vi "Add PV - NT Enum (Reference).vi"(5 "is read only? (F)":bool, 6 "initial timestamp":timestamp, 7 "PV name":string, 8 "error in (no error)":errorcluster, 10 "ref":refnum<vi>, 11 "Server in":refnum<class "Server.lvclass">) -> (0 "error out":errorcluster, 2 "ref out":refnum<vi>, 3 "Server out":refnum<class "Server.lvclass">)   [LabVIEW 2020, in "PV Access.lvlib" / "PVA Server.lvlib" / "Server.lvclass"]
uses:
  Server.lvclass
  Server.lvclass/Server.ctl
  PV Data/NT Enum/NT Enum.lvclass
  Source/Source.lvclass
  PV Data/PV Data.lvlib
  PV Data/NT Enum/Create - Enum.vi
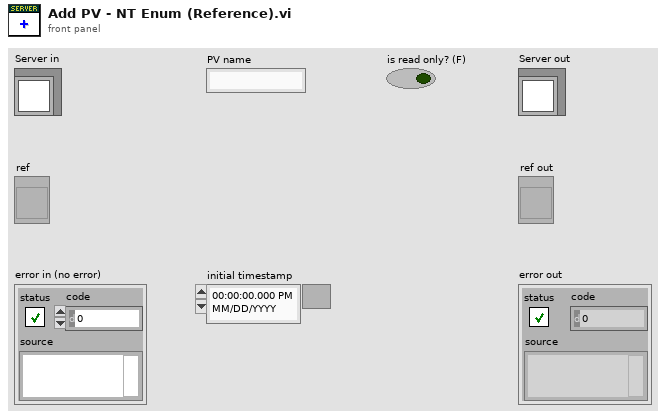
[diagram p1: front panel]
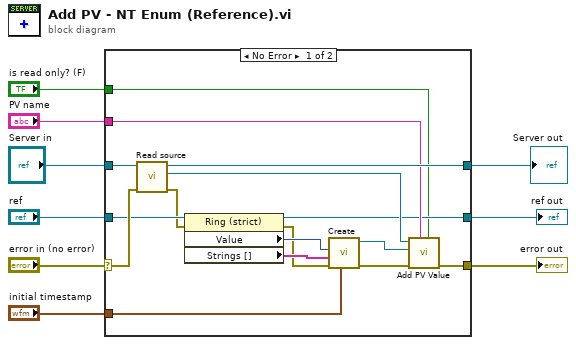
[diagram p0: block diagram]
diagram:
  n1 = case shown="No Error" "error in (no error)" {
    selector: "error in (no error)" -> [w21 w28]
    tunnel: [w20 w28] -> w8
    tunnel: [w24 w27] -> w6
    tunnel: "Server in" -> [w25 w27]
    tunnel: "PV name" -> [w22 _]
    tunnel: "initial timestamp" -> [w17 _]
    tunnel: "ref" -> [w16 w26]
    tunnel: [w11 w26] -> w2
    tunnel: "is read only? (F)" -> [w10 _]
    frame No Error {
      n2 = call "Read source.vi"("error in (no error)"=w21, "Server in"=w25) -> ("error out"=w15:errorcluster, "Source"=w23:refnum<class "Source.lvclass">, "Server out"=w24:refnum<class "Server.lvclass">)  [unwired: 7 in]
      n3 = property class="Ring (strict)"(reference=w16, error in=w15) -> (reference out=w11:refnum<vi>, error out=w12:errorcluster, "Value"=w14:u16, "Strings []"=w13:string[])
      n4 = call-poly "Create.vi"("initial timestamp"=w17, "error in (no error)"=w12, "choices"=w13, "initial index"=w14) -> ("error out"=w19:errorcluster, "NT Enum out"=w18:refnum<class "NT Enum.lvclass">)  [unwired: 6 in]
      n5 = call "Add PV Value.vi"("is read only? (F)"=w10, "PV name"=w22, "error in"=w19, "value in"=w18, "Source in"=w23) -> ("error out"=w20:errorcluster)  [unwired: 4 in, 2 out]
    }
    frame Error {
    }
  }
  "error out" <- w8
  "Server out" <- w6
  "ref out" <- w2
